vi "Design a Filter Step by Step.vi"() -> ()   [LabVIEW 2023]
doc: "Demonstrates a typical digital design process that you can follow when using the LabVIEW Digital Filter Design Toolkit to design and use floating-point and fixed-point filters. Run the VI and follow the instructions to start the digital filter design process.\n\n<B>Tip:</B> You can display the context help information for each option on the <B>Design a Filter Step by Step</B> window by pressing the <Ctrl-H> keys."
panel:
  in  "Fixed-Point Modeling & Simulation":bool
  in  "Structure Selection & Coefficients Quantization":bool
  in  "Floating-Point Filtering":bool
  in  "Floating-Point Filter Design & Analysis":bool
  in  "Deployment to NI-RIO Device":bool
  in  "Fixed-Point Code Generation":bool
  out "arrow3":bool
  out "arrow4":bool
  out "arrow2":bool
  out "arrow1":bool
  in  "step":i32=-1
  in  "Stop":bool
  # "Typical Digital Filter Design Process"
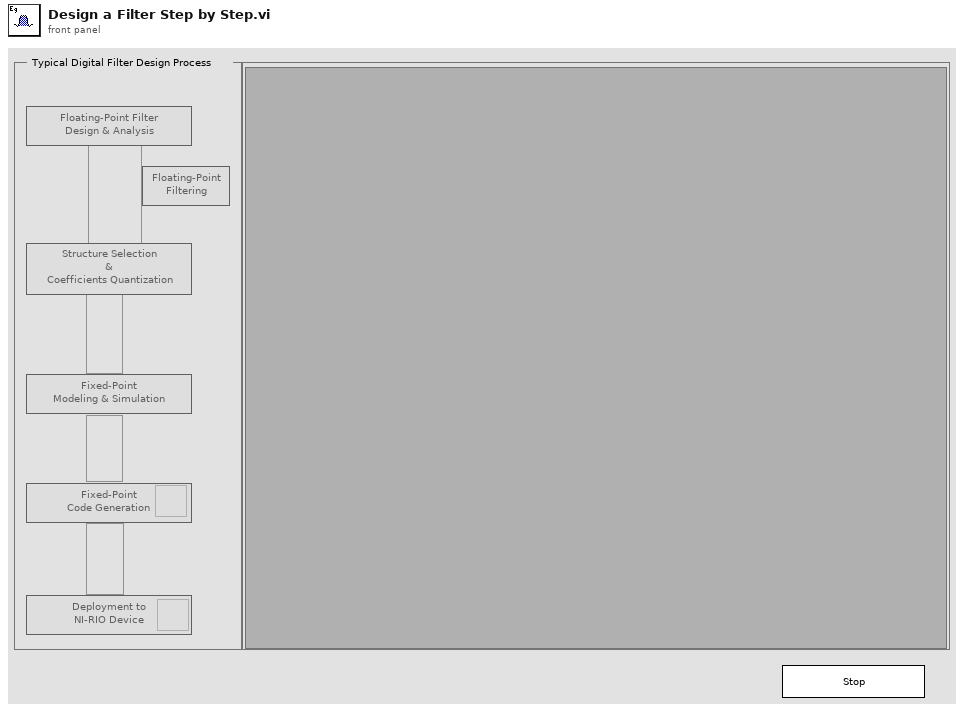
[diagram p1: front panel]
types:
  T1 = typedef "NI_DigFilterLicensed.lvlib/DFD Filter Obj.ctl" = cluster{"mSRate_Fs":dbl, "mSRate_Version":string, "mSRate_Comments":string, "mSRate_OrgCoef":T2, "mSRate_CurCoef":T2, "mSRate_Quantized?":bool, "mSRate_QCoef":T2, "mSRate_QSettings":T4[], "mSRate_Order":i32, "mSRate_Scaling":cluster{"mSRate_ScaleByPowerOf2?":bool, "mSRate_ScaleType":T6}}
  T2 = typedef "NI_DigFilterLicensed.lvlib/DFD Filter Coef.ctl" = cluster{"type":T3, "gain":dbl, "coef a (k)":dbl[], "coef b (v)":dbl[]}
  T3 = typedef "NI_DigFilterLicensed.lvlib/DFD Filter Structure Type Selector.ctl" = enum16{"Undefined", "FIR Direct Form", "FIR Direct Form Transposed", "FIR Symmetric", "FIR Antisymmetric", "IIR Direct Form I", "IIR Direct Form I Transposed", "IIR Direct Form II", "IIR Direct Form II Transposed", "IIR Cascaded Second Order Sections Form I", "IIR Cascaded Second Order Sections Form I Transposed", "IIR Cascaded Second Order Sections Form II", "IIR Cascaded Second Order Sections Form II Transposed", "Lattice Allpass (basic sections)", "Lattice Allpass (one multiplier sections)", "Lattice Allpass (normalized sections)", "Lattice AR (basic sections)", "Lattice AR (one multiplier sections)", "Lattice AR (normalized sections)", "Lattice MA (minimum phase)", "Lattice MA (maximum phase)", "Lattice ARMA (basic sections)", "Lattice ARMA (one multiplier sections)", "Lattice ARMA (normalized sections)"}
  T4 = typedef "NI_DigFilterLicensed.lvlib/dfd_Internal Quantization Settings.ctl" = cluster{"source":T5, "wl":i16, "iwl":i16, "overflow mode":enum16{"Saturation", "Wrap"}, "rounding mode":enum16{"Nearest", "Truncation"}, "signed?":bool}
  T5 = typedef "NI_DigFilterLicensed.lvlib/dfd_Internal Quantization Srcs.ctl" = u16
  T6 = typedef "NI_DigFilterLicensed.lvlib/DFD Coef Norm Type.ctl" = enum16{"No Norm", "Time Domain 1-Norm", "Time Domain 2-Norm", "Time Domain Inf-Norm"}
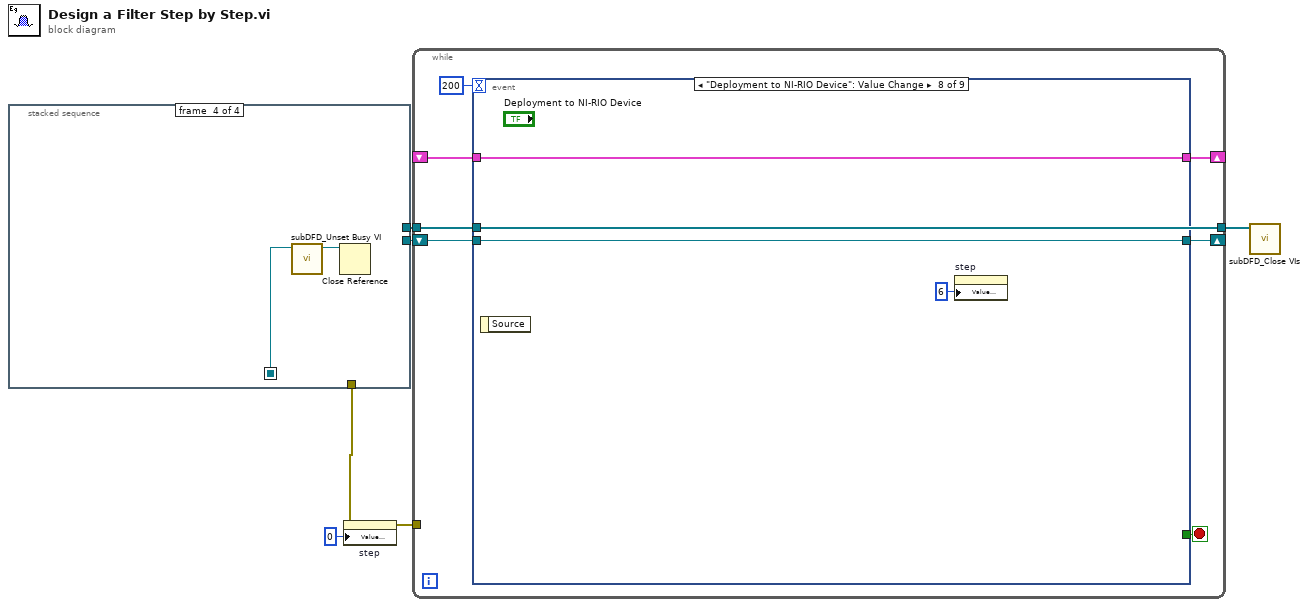
[diagram p0: block diagram]
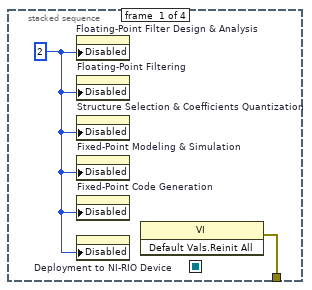
[diagram p2: hidden frame]
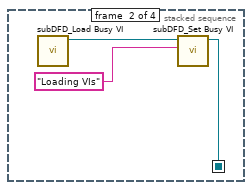
[diagram p3: hidden frame]
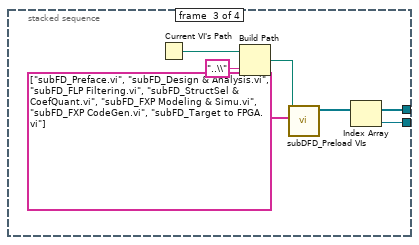
[diagram p4: hidden frame]
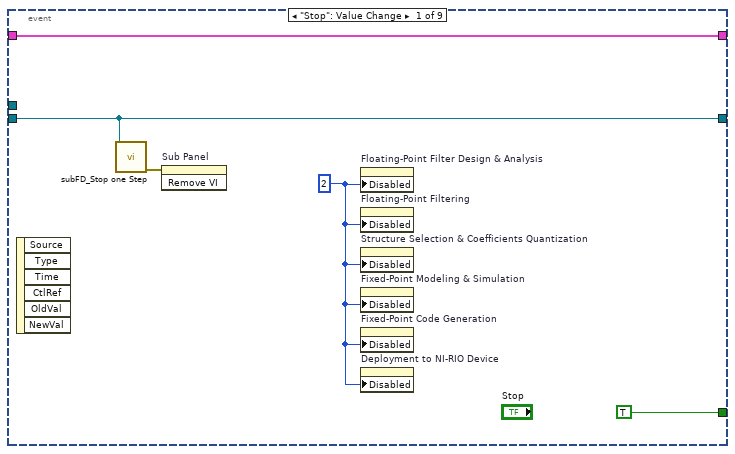
[diagram p5: hidden frame]
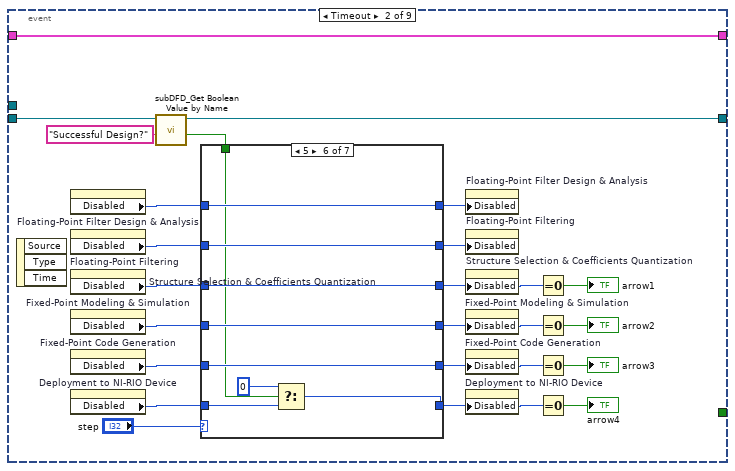
[diagram p6: hidden frame]
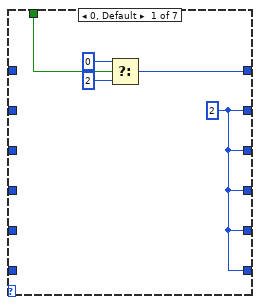
[diagram p7: hidden frame]
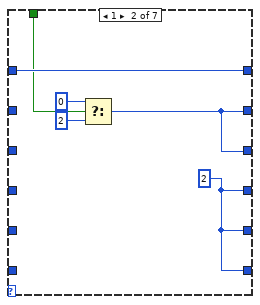
[diagram p8: hidden frame]
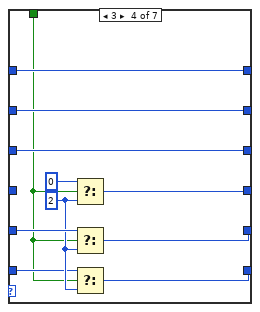
[diagram p10: hidden frame]
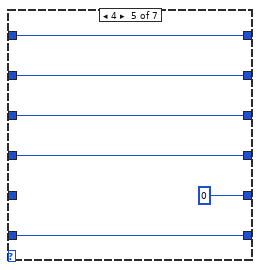
[diagram p11: hidden frame]
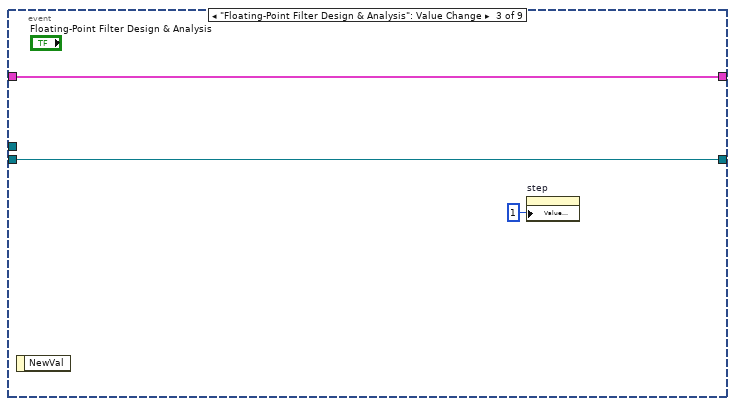
[diagram p13: hidden frame]
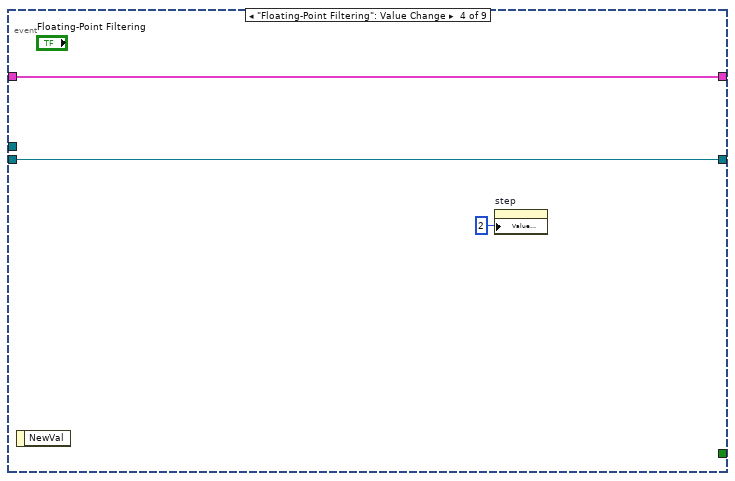
[diagram p14: hidden frame]
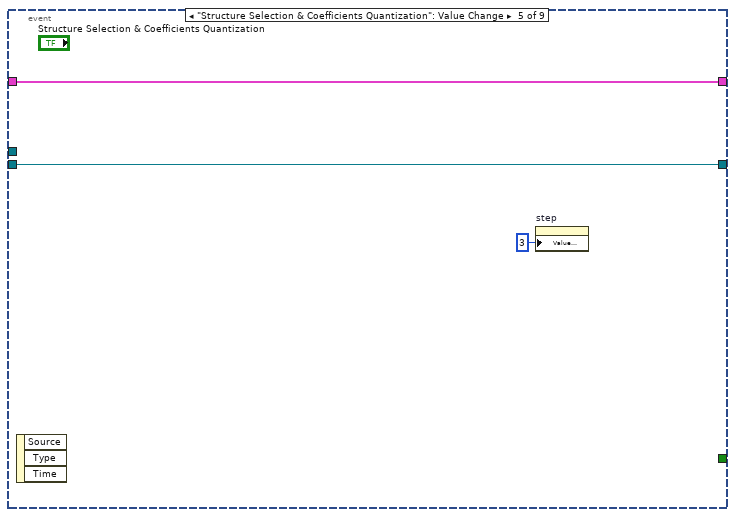
[diagram p15: hidden frame]
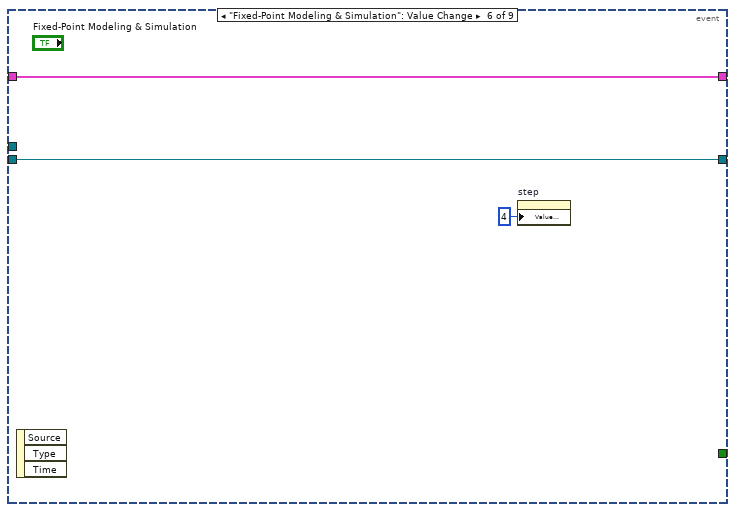
[diagram p16: hidden frame]
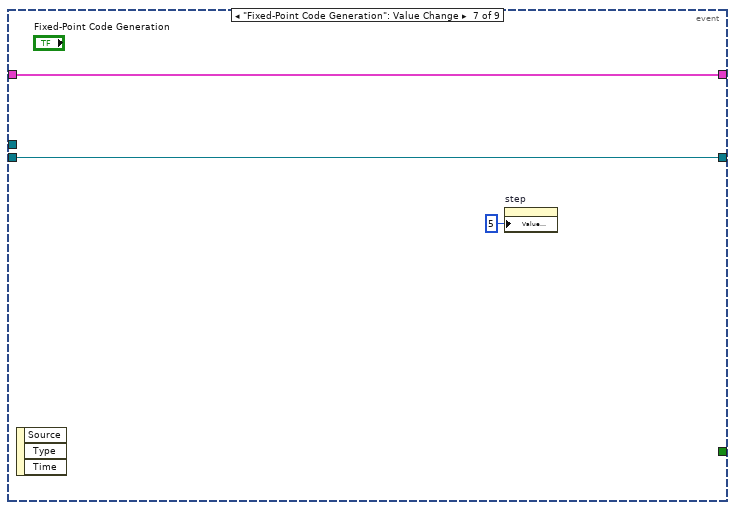
[diagram p17: hidden frame]
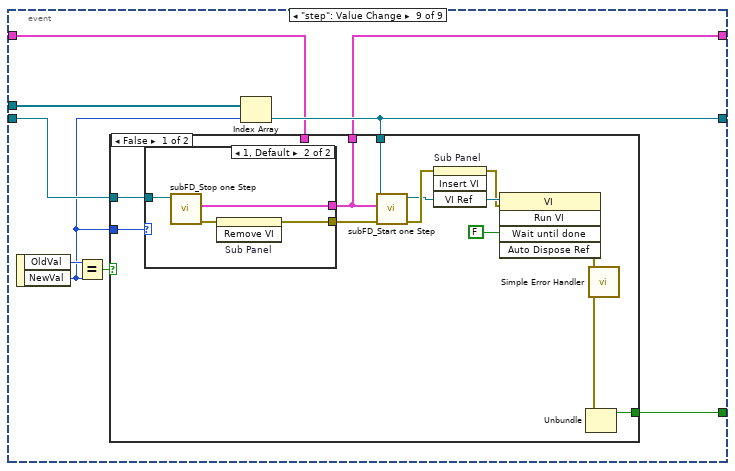
[diagram p18: hidden frame]
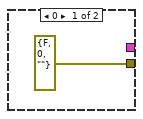
[diagram p19: hidden frame]
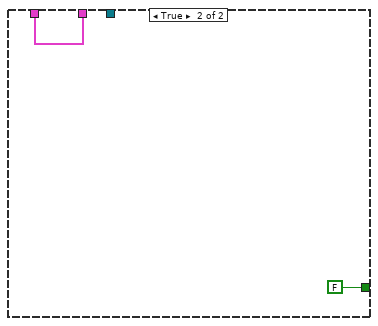
[diagram p20: hidden frame]
diagram:
  n1 = stacked-sequence {
    seq-local: [_ w11 _ _] -> [_ _ _ w19]
    tunnel: [_ _ w17 _] -> w6
    tunnel: [_ _ w16 _] -> w5
    tunnel: [w7 _ _ _] -> w1
    frame #0 {
      w8 = u8 2 ("Disabled")
      n2 = property on="Floating-Point Filter Design & Analysis" class="Bool"("Disabled"=w8) -> ()  [unwired: 2 in, 2 out]
      n3 = property on="Floating-Point Filtering" class="Bool"("Disabled"=w8) -> ()  [unwired: 2 in, 2 out]
      n4 = property on="Structure Selection & Coefficients Quantization" class="Bool"("Disabled"=w8) -> ()  [unwired: 2 in, 2 out]
      n5 = property on="Fixed-Point Modeling & Simulation" class="Bool"("Disabled"=w8) -> ()  [unwired: 2 in, 2 out]
      n6 = property on="Fixed-Point Code Generation" class="Bool"("Disabled"=w8) -> ()  [unwired: 2 in, 2 out]
      n7 = property on="Deployment to NI-RIO Device" class="Bool"("Disabled"=w8) -> ()  [unwired: 2 in, 2 out]
      n8 = invoke class="VI" method="Default Vals.Reinit All"() -> (error out=w7:errorcluster)  [unwired: 3 in, 2 out]
    }
    frame #1 {
      n9 = call <vilib>:"subDFD_Load Busy VI.vi"() -> ("Busy vi reference"=w9:refnum<vi>)  [unwired: 11 out]
      n10 = call <vilib>:"subDFD_Set Busy VI.vi"("busy task"="Loading VIs" ("control name"), "Busy vi reference"=w9) -> ("dup Busy vi reference"=w11:refnum<vi>)  [unwired: 1 in, 8 out]
    }
    frame #2 {
      n11 = Current VI's Path() -> (path=w15:path)
      n12 = Build Path(base path=w15, name or relative path="..\\") -> (appended path=w13:path)
      n13 = call "subDFD_Preload VIs.vi"("VI names"=string[] ["subFD_Preface.vi", "subFD_Design & Analysis.vi", "subFD_FLP Filtering.vi", "subFD_StructSel & CoefQuant.vi", "subFD_FXP Modeling & Simu.vi", "subFD_FXP CodeGen.vi", "subFD_Target to FPGA.vi"], "source folder"=w13) -> ("all VIs refs"=w16:refnum<vi>[])  [unwired: 1 in, 8 out]
      n14 = Index Array(array=w16) -> (element=w17:refnum<vi>)  [unwired: 1 in]
    }
    frame #3 {
      n15 = call <vilib>:"subDFD_Unset Busy VI.vi"("Busy vi reference"=w19) -> ("dup Busy vi reference"=w18:refnum<vi>)  [unwired: 1 in, 9 out]
      n16 = Close Reference(reference=w18) -> ()  [unwired: 1 in, 1 out]
    }
  }
  n17 = property on="step" class="DigNum (strict)"(error in=w1, "Value (Signaling)"=0) -> (error out=w3:errorcluster)  [unwired: 1 in, 1 out]
  n18 = while {
    shift-right: [w23] -> _
    shift-left: w6 -> [w24]
    shift-right: [w22] -> _
    shift-left: _ -> [w21]
    tunnel: w5 -> [w20]
    tunnel: w3 -> [_]
    tunnel: [w20] -> w2
    stop <- w26 stop-if-true
    n19 = event shown="[7] \"Deployment to NI-RIO Device\": Value Change" {
      selector: _ -> [_ _ _ _ _ _ _ _ _]
      dyn-events: _ -> [_ _ _ _ _ _ _ _ _]
      timeout: 200 -> [_ _ _ _ _ _ _ _ _]
      tunnel: [TRUE ("OK") _ _ _ _ _ _ _ w122] -> w26
      tunnel: w24 -> [w29 w53 w104 w107 w109 w113 w116 w119 w127]
      tunnel: [w29 w51 w104 w107 w109 w113 w116 w119 w125] -> w23
      tunnel: [w31 w50 w105 w108 w111 w114 w117 w120 w124] -> w22
      tunnel: w21 -> [w31 w50 w105 w108 w111 w114 w117 w120 w123]
      tunnel: w20 -> [_ _ _ _ _ _ _ _ w121]
      event "Stop": Value Change {
        w27 = u8 2 ("Disabled")
        n20 = event-data() -> ()  [unwired: 7 out]
        n21 = call "subFD_Stop one Step.vi"("vi refnum in"=w29) -> ("error out"=w30:errorcluster)  [unwired: 1 in, 9 out]
        n22 = invoke on="Sub Panel" class="SubPnl" method="Remove VI"(error in=w30) -> ()  [unwired: 2 in, 3 out]
        n23 = property on="Floating-Point Filter Design & Analysis" class="Bool"("Disabled"=w27) -> ()  [unwired: 2 in, 2 out]
        n24 = property on="Floating-Point Filtering" class="Bool"("Disabled"=w27) -> ()  [unwired: 2 in, 2 out]
        n25 = property on="Structure Selection & Coefficients Quantization" class="Bool"("Disabled"=w27) -> ()  [unwired: 2 in, 2 out]
        n26 = property on="Fixed-Point Modeling & Simulation" class="Bool"("Disabled"=w27) -> ()  [unwired: 2 in, 2 out]
        n27 = property on="Fixed-Point Code Generation" class="Bool"("Disabled"=w27) -> ()  [unwired: 2 in, 2 out]
        n28 = property on="Deployment to NI-RIO Device" class="Bool"("Disabled"=w27) -> ()  [unwired: 2 in, 2 out]
      }
      event Timeout {
        n29 = event-data() -> ()  [unwired: 4 out]
        n30 = property on="Floating-Point Filter Design & Analysis" class="Bool"() -> ("Disabled"=w48:u8)  [unwired: 2 in, 2 out]
        n31 = property on="Floating-Point Filtering" class="Bool"() -> ("Disabled"=w47:u8)  [unwired: 2 in, 2 out]
        n32 = property on="Structure Selection & Coefficients Quantization" class="Bool"() -> ("Disabled"=w46:u8)  [unwired: 2 in, 2 out]
        n33 = property on="Fixed-Point Modeling & Simulation" class="Bool"() -> ("Disabled"=w45:u8)  [unwired: 2 in, 2 out]
        n34 = property on="Fixed-Point Code Generation" class="Bool"() -> ("Disabled"=w44:u8)  [unwired: 2 in, 2 out]
        n35 = property on="Deployment to NI-RIO Device" class="Bool"() -> ("Disabled"=w43:u8)  [unwired: 2 in, 2 out]
        n36 = call "subDFD_Get Boolean Value by Name.vi"("Control Name"="Successful Design?" ("control name"), "vi reference in"=w53) -> ("Boolean"=w40:bool, "vi reference out"=w51:refnum<vi>)  [unwired: 1 in, 7 out]
        n37 = case shown="5" "step" {
          tunnel: w48 -> [_ w63 w70 w81 w87 w96 w102]
          tunnel: w47 -> [_ _ w69 w80 w86 w95 w101]
          tunnel: w46 -> [_ _ w68 w79 w85 w94 w100]
          tunnel: w45 -> [_ _ w67 _ w84 w93 w99]
          tunnel: w44 -> [_ _ w66 w76 _ w92 w98]
          tunnel: w43 -> [_ _ w65 w74 w82 w89 w97]
          tunnel: [w55 w63 w70 w81 w87 w96 w102] -> w42
          tunnel: [w58 w60 w69 w80 w86 w95 w101] -> w41
          tunnel: [w58 w60 w68 w79 w85 w94 w100] -> w39
          tunnel: [w58 w64 w67 w77 w84 w93 w99] -> w37
          tunnel: [w58 w64 w66 w73 u8 0 ("Disabled") w92 w98] -> w35
          tunnel: [w58 w64 w65 w72 w82 w88 w97] -> w33
          tunnel: w40 -> [w57 w59 _ w71 _ w91 _]
          frame 0, Default {
            w58 = u8 2
            n38 = Select(t=u8 0, s=w57, f=u8 2) -> (s? t:f=w55:u8)
          }
          frame 1 {
            w64 = u8 2
            n39 = Select(t=u8 0, s=w59, f=u8 2) -> (s? t:f=w60:u8)
          }
          frame 2 {
          }
          frame 3 {
            w75 = u8 2 ("f")
            n40 = Select(t=u8 0, s=w71, f=w75) -> (s? t:f=w77:u8)
            n41 = Select(t=w76, s=w71, f=w75) -> (s? t:f=w73:u8)
            n42 = Select(t=w74, s=w71, f=w75) -> (s? t:f=w72:u8)
          }
          frame 4 {
          }
          frame 5 {
            n43 = Select(t=u8 0 ("Disabled"), s=w91, f=w89) -> (s? t:f=w88:u8)
          }
          frame 6 {
          }
        }
        n44 = property on="Floating-Point Filter Design & Analysis" class="Bool"("Disabled"=w42) -> ()  [unwired: 2 in, 2 out]
        n45 = property on="Floating-Point Filtering" class="Bool"("Disabled"=w41) -> ()  [unwired: 2 in, 2 out]
        n46 = property on="Structure Selection & Coefficients Quantization" class="Bool"("Disabled"=w39) -> ()  [unwired: 2 in, 2 out]
        n47 = property on="Fixed-Point Modeling & Simulation" class="Bool"("Disabled"=w37) -> ()  [unwired: 2 in, 2 out]
        n48 = property on="Fixed-Point Code Generation" class="Bool"("Disabled"=w35) -> ()  [unwired: 2 in, 2 out]
        n49 = property on="Deployment to NI-RIO Device" class="Bool"("Disabled"=w33) -> ()  [unwired: 2 in, 2 out]
        n50 = Equal To 0?(x=w39) -> (x = 0?=→"arrow1":bool)
        n51 = Equal To 0?(x=w37) -> (x = 0?=→"arrow2":bool)
        n52 = Equal To 0?(x=w35) -> (x = 0?=→"arrow3":bool)
        n53 = Equal To 0?(x=w33) -> (x = 0?=→"arrow4":bool)
      }
      event "Floating-Point Filter Design & Analysis": Value Change {
        n54 = event-data() -> ()  [unwired: 2 out]
        n55 = property on="step" class="DigNum (strict)"("Value (Signaling)"=1) -> ()  [unwired: 2 in, 2 out]
      }
      event "Floating-Point Filtering": Value Change {
        n56 = event-data() -> ()  [unwired: 2 out]
        n57 = property on="step" class="DigNum (strict)"("Value (Signaling)"=2) -> ()  [unwired: 2 in, 2 out]
      }
      event "Structure Selection & Coefficients Quantization": Value Change {
        n58 = event-data() -> ()  [unwired: 4 out]
        n59 = property on="step" class="DigNum (strict)"("Value (Signaling)"=3) -> ()  [unwired: 2 in, 2 out]
      }
      event "Fixed-Point Modeling & Simulation": Value Change {
        n60 = event-data() -> ()  [unwired: 4 out]
        n61 = property on="step" class="DigNum (strict)"("Value (Signaling)"=4) -> ()  [unwired: 2 in, 2 out]
      }
      event "Fixed-Point Code Generation": Value Change {
        n62 = event-data() -> ()  [unwired: 4 out]
        n63 = property on="step" class="DigNum (strict)"("Value (Signaling)"=5) -> ()  [unwired: 2 in, 2 out]
      }
      event "Deployment to NI-RIO Device": Value Change {
        n64 = event-data() -> ()  [unwired: 2 out]
        n65 = property on="step" class="DigNum (strict)"("Value (Signaling)"=6) -> ()  [unwired: 2 in, 2 out]
      }
      event "step": Value Change {
        n66 = event-data() -> ("OldVal"=w129:i32, "NewVal"=w126:i32)  [unwired: 1 out]
        n67 = Equal?(x=w129, y=w126) -> (x = y?=w128:bool)
        n68 = Index Array(array=w121, index=w126) -> (element=w125:refnum<vi>)
        n69 = case shown="False" w128 {
          tunnel: w127 -> [w140 _]
          tunnel: w126 -> [w139 _]
          tunnel: w125 -> [w137 _]
          tunnel: [w130 w147] -> w124
          tunnel: w123 -> [_ w147]
          tunnel: [w131 FALSE ("status")] -> w122
          frame False {
            n70 = case shown="1, Default" w139 {
              tunnel: w140 -> [_ w145]
              tunnel: [_ w143] -> w130
              tunnel: [errorcluster {"status"=FALSE, "code"=0, "source"=""} ("error out") w142] -> w138
              frame 0 {
              }
              frame 1, Default {
                n71 = call "subFD_Stop one Step.vi"("vi refnum in"=w145) -> ("error out"=w144:errorcluster, "filter out"=w143:T1)  [unwired: 1 in, 8 out]
                n72 = invoke on="Sub Panel" class="SubPnl" method="Remove VI"(error in=w144) -> (error out=w142:errorcluster)  [unwired: 2 in, 2 out]
              }
            }
            n73 = call "subFD_Start one Step.vi"("error in (no error)"=w138, "filter in"=w130, "vi refnum in"=w137) -> ("error out"=w136:errorcluster, "vi refnum out"=w134:refnum<vi>)  [unwired: 7 out]
            n74 = invoke on="Sub Panel" class="SubPanel" method="Insert VI"(error in=w136, "VI Ref"=w134) -> (error out=w133:errorcluster)  [unwired: 2 in, 3 out]
            n75 = invoke class="VI" method="Run VI"(reference=w134, error in=w133, "Wait until done"=FALSE) -> (error out=w132:errorcluster)  [unwired: 2 in, 4 out]
            n76 = Unbundle(w132) -> ("status"=w131:bool)  [unwired: 2 out]
            n77 = call <vilib>:"Simple Error Handler.vi"("error in (no error)"=w132) -> ()  [unwired: 1 in, 8 out]
          }
          frame True {
          }
        }
      }
    }
  }
  n78 = call "subDFD_Close VIs.vi"("all VIs refs"=w2) -> ()  [unwired: 1 in, 10 out]
